vi "tearDown.vi"(8 "error in (no error)":errorcluster, 11 "reference in":refnum<class "SLSC Switch Scripting Unit Tests.lvclass">) -> (0 "error out":errorcluster, 3 "reference out":refnum<class "SLSC Switch Scripting Unit Tests.lvclass">)   [LabVIEW 2017, in "SLSC Switch Scripting Unit Tests.lvclass"]
doc: "tearDown runs after the test method has completed. Use this method to clean up any operations or references that were opened by setUp or the test method. Unit tests should be independent of other unit tests so this VI should ensure that the next test can run in a 'clean' test environment."
uses:
  SLSC Switch Scripting Unit Tests.lvclass
  SLSC Switch Scripting Unit Tests.lvclass/SLSC Switch Scripting Unit Tests.ctl
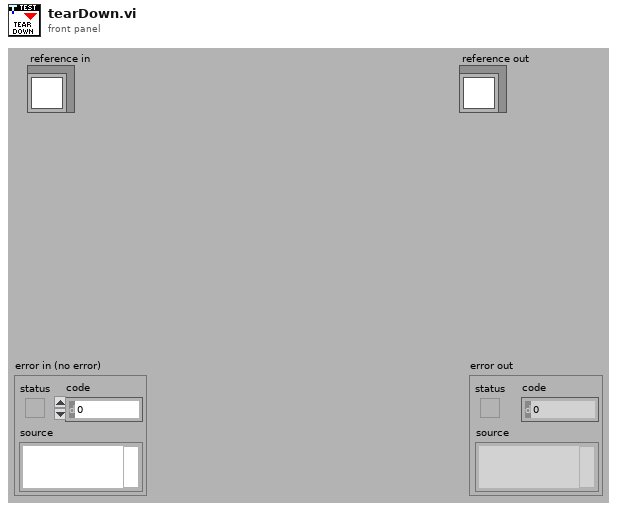
[diagram p1: front panel]
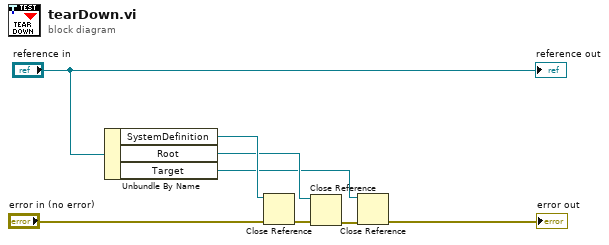
[diagram p0: block diagram]
diagram:
  n1 = Unbundle By Name("reference in") -> ("SystemDefinition"=w5:refnum<k24>, "Root"=w4:refnum<k24>, "Target"=w3:refnum<k24>)
  n2 = Close Reference(reference=w5, error in (no error)="error in (no error)") -> (error out=w7:errorcluster)
  n3 = Close Reference(reference=w4, error in (no error)=w7) -> (error out=w6:errorcluster)
  n4 = Close Reference(reference=w3, error in (no error)=w6) -> (error out=→"error out":errorcluster)
  "reference out" <- "reference in"
